vi "module for color detection.vi"() -> ()   [LabVIEW 2018]
uses:
  <vilib>/userdefined/High Color/IMAQdx.ctl
  <vilib>/vision/driver/NI_Vision_Acquisition_Software.lvlib
  <vilib>/vision/NI_Vision_Development_Module.lvlib
panel:
  out "green 2":bool
  out "Image":T1(plugin-control)
  out "yellow":bool
  out "black":bool
  out "red 2":bool
  out "blue 2":bool
  in  "Color Sensitivity":u32(ring) items=["Low", "Medium", "High"]
  out "Color Spectrum":dbl[](array[numeric]) format="%.2f"
  in  "stop":bool
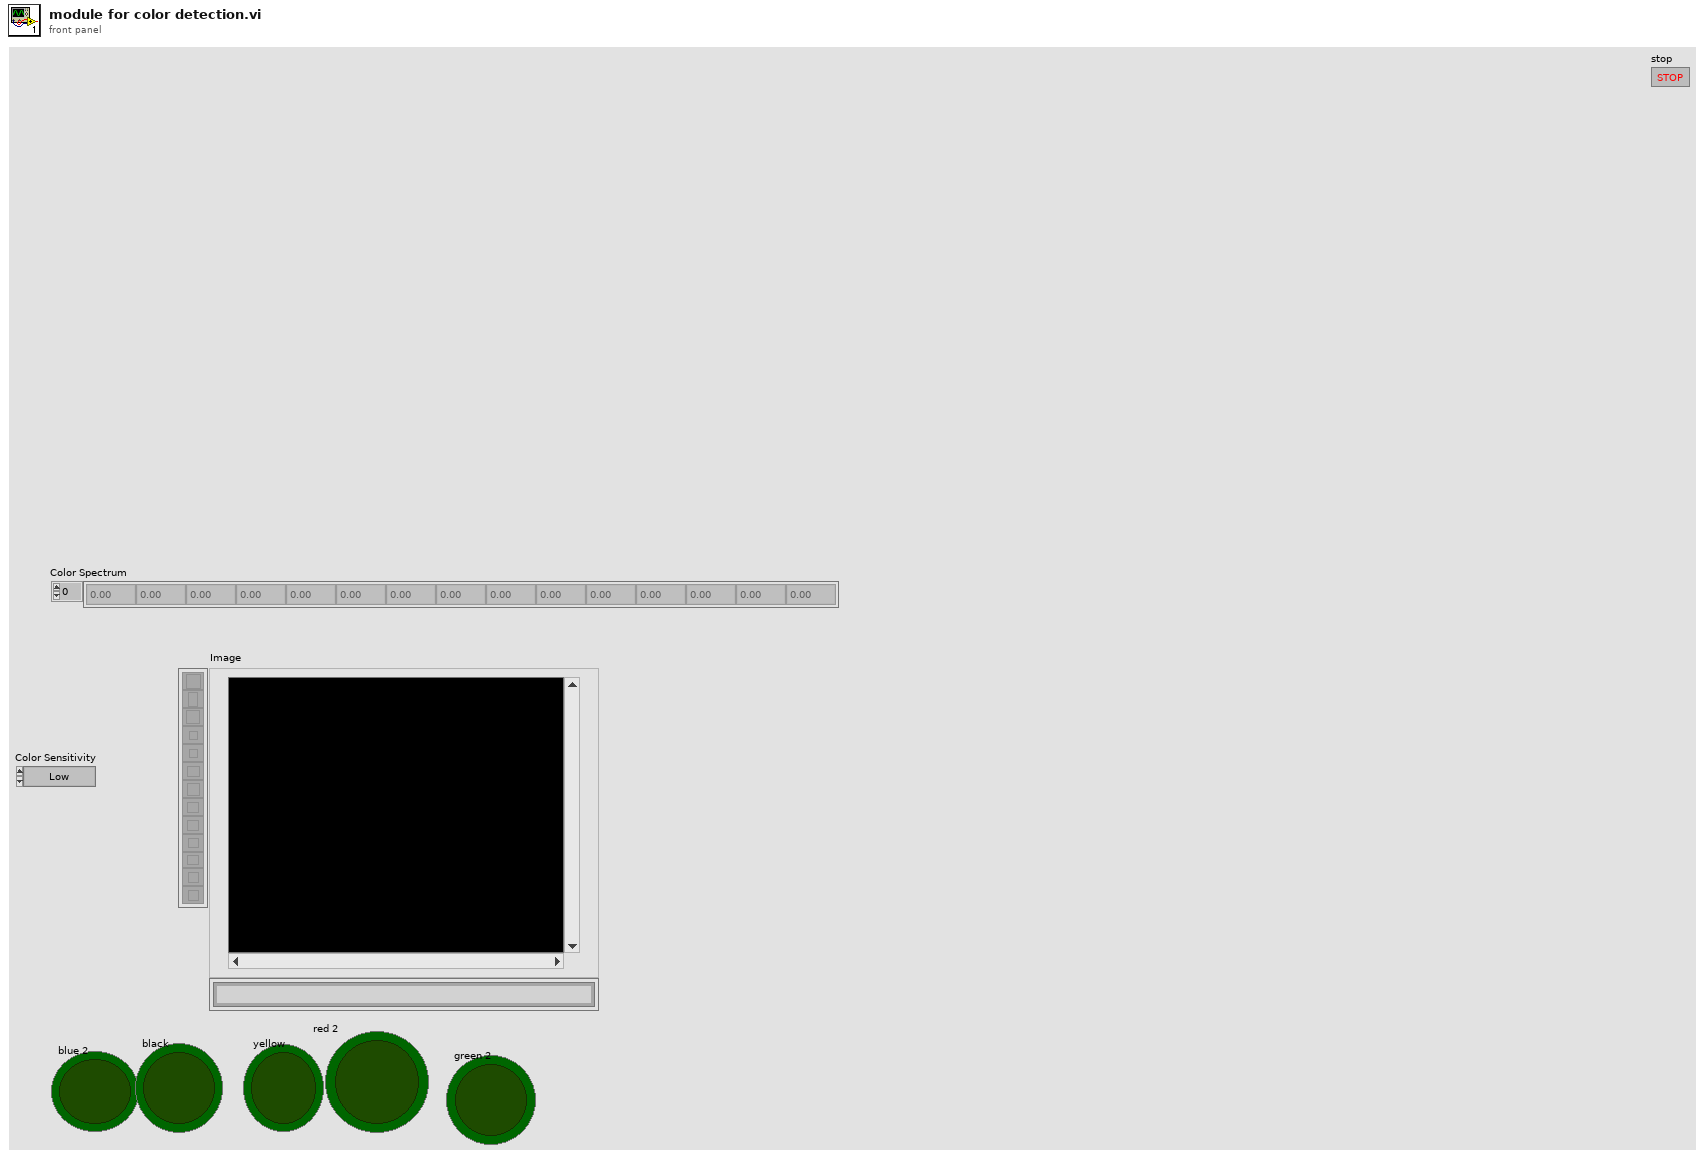
[diagram p1: front panel]
types:
  T1 = typedef "IMAQ Image.ctl" = refnum<image>
  T2 = typedef "IMAQdx.ctl" = refnum<k21>
  T3 = cluster{"Global Rectangle":i32[], "Contours":cluster{"Contour Type":u32, "ROI Type":u32, "Points":i32[]}[]}
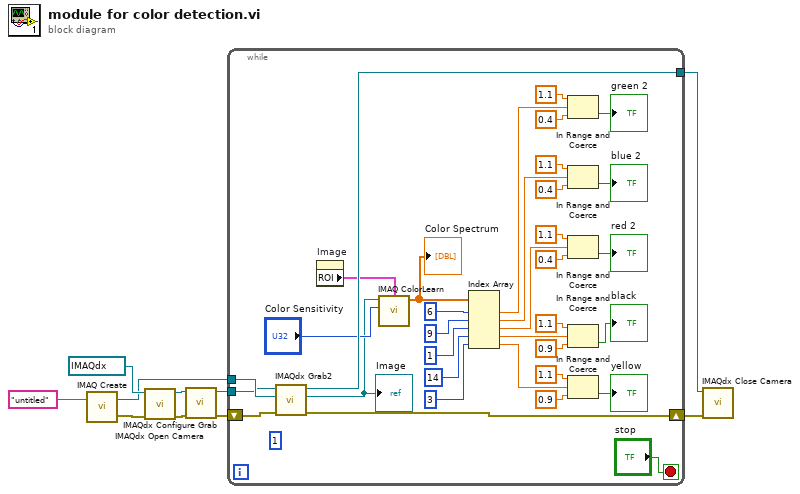
[diagram p0: block diagram]
diagram:
  n1 = call "IMAQ Create"("Image Name"="untitled") -> ("New Image"=w3:T1, "error out"=w10:errorcluster)  [unwired: 4 in]
  n2 = call <vilib>:"IMAQdx Open Camera.vi"("error in"=w10, "Session In"=T2 "cam0") -> ("error out"=w8:errorcluster, "Session Out"=w9:T2)  [unwired: 8 in]
  n3 = call <vilib>:"IMAQdx Configure Grab.vi"("error in"=w8, "Session In"=w9) -> ("error out"=w5:errorcluster, "Session Out"=w2:T2)  [unwired: 8 in]
  n4 = while {
    shift-right: [w43] -> w4
    shift-left: w5 -> [w44]
    tunnel: w3 -> [w42]
    tunnel: w2 -> [w41]
    tunnel: [w40] -> w1
    stop <- "stop" stop-if-true
    (unwired) 1
    n5 = call <vilib>:"IMAQdx Grab2.vi"("error in"=w44, "Image In"=w42, "Session In"=w41) -> ("error out"=w43:errorcluster, "Image Out"=w15:T1, "Session Out"=w40:T2)  [unwired: 5 in, 1 out]
    "Image" <- w15
    n6 = property on="Image" class="ImageControl"() -> ("ROI"=w14:T3)  [unwired: 2 in, 2 out]
    n7 = call "IMAQ ColorLearn"("ROI Descriptor"=w14, "Image"=w15, "Color Sensitivity"="Color Sensitivity") -> ("Color Spectrum"=w36:dbl[])  [unwired: 5 in, 1 out]
    "Color Spectrum" <- w36
    n8 = Index Array(array=w36, index #1=6 ("index"), index #2=9 ("index"), index #3=1 ("index"), index #4=14 ("index"), index #5=3 ("index")) -> (element #1=w13:dbl, element #2=w30:dbl, element #3=w27:dbl, element #4=w24:dbl, element #5=w22:dbl)
    n9 = In Range and Coerce(upper limit=1.1, x=w13, lower limit=0.4 ("upper limit")) -> (In Range?=→"green 2":bool)  [unwired: 1 out]
    n10 = In Range and Coerce(upper limit=1.1, x=w30, lower limit=0.4) -> (In Range?=→"blue 2":bool)  [unwired: 1 out]
    n11 = In Range and Coerce(upper limit=1.1, x=w27, lower limit=0.4 ("element")) -> (In Range?=→"red 2":bool)  [unwired: 1 out]
    n12 = In Range and Coerce(upper limit=1.1, x=w24, lower limit=0.9) -> (In Range?=→"black":bool)  [unwired: 1 out]
    n13 = In Range and Coerce(upper limit=1.1, x=w22, lower limit=0.9) -> (In Range?=→"yellow":bool)  [unwired: 1 out]
  }
  n14 = call <vilib>:"IMAQdx Close Camera.vi"("error in"=w4, "Session In"=w1) -> ()  [unwired: 9 in, 1 out]
